vi "Atto DRY Interface get4K Stage Temperature.vi"(8 "error in (no error)":errorcluster, 11 "_4KStageTemperatureK":sgl) -> (0 "error out":errorcluster, 2 "function return":i32, 3 "_4KStageTemperatureK out":sgl)   [LabVIEW 2016, in "attoDRYLib.lvlib"]
doc: "int32_t __cdecl AttoDRY_Interface_get4KStageTemperature(\n float *_4KStageTemperatureK);"
uses:
  <userlib>/attoDRYLib/attoDRYLib.lvlib
  <userlib>/attoDRYLib/attoDRYLib.dll
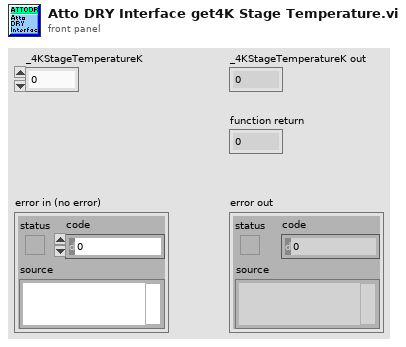
[diagram p1: front panel]
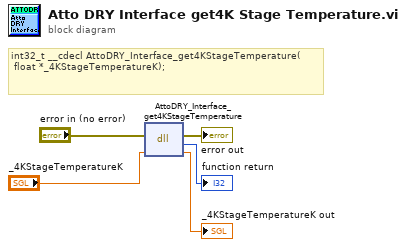
[diagram p0: block diagram]
diagram:
  # "int32_t __cdecl AttoDRY_Interface_get4KStageTemperature(\n\tfloat *_4KStageTemperatureK);"
  n1 = dll-call lib="C:/Program Files (x86)/National Instruments/LabVIEW 2016/user.lib/attoDRYLib/attoDRYLib.*" fn="AttoDRY_Interface_get4KStageTemperature"(error in="error in (no error)", "_4KStageTemperatureK"="_4KStageTemperatureK") -> (error out=→"error out":errorcluster, →"function return":i32, "_4KStageTemperatureK"=→"_4KStageTemperatureK out":sgl)  [unwired: 2 in, 1 out]
